vi "Delay.vi"(8 "error in (no error)":errorcluster, 11 "VISA resource name":refnum<visa-resource-name>) -> (0 "error out":errorcluster, 3 "VISA resource name out":refnum<visa-resource-name>)   [LabVIEW 2022 SP3]
panel:
  # "ms"
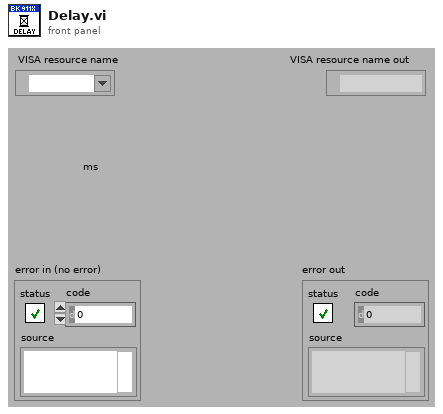
[diagram p1: front panel]
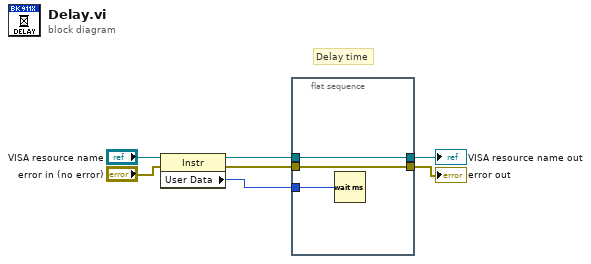
[diagram p0: block diagram]
diagram:
  # "Delay time"
  n1 = property class="Instr"(reference="VISA resource name", error in="error in (no error)") -> (reference out=w4:refnum<visa-resource-name>, error out=w3:errorcluster, "User Data"=w5:u32)
  n2 = flat-sequence {
    tunnel: w5 -> [w10]
    tunnel: [w9] -> w7
    tunnel: w4 -> [w9]
    tunnel: [w8] -> w6
    tunnel: w3 -> [w8]
    frame #0 {
      n3 = Wait (ms)(milliseconds to wait=w10) -> ()  [unwired: 1 out]
    }
  }
  "VISA resource name out" <- w7
  "error out" <- w6
